vi "EV03全局.vi"() -> ()   [LabVIEW 2013]
panel:
  out "Stop":bool
  out "判定测量值":bool
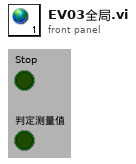
[diagram p1: front panel]
diagram:
